vi "SwerveMain.vi"   [LabVIEW 2018]
uses:
  <vilib>/Rock Robotics/WPI/ThirdParty/Phoenix-LabVIEW/Motor Controller/Controls/CTRE_Phoenix_MotorControl_ControlMode.ctl
  <vilib>/Rock Robotics/Network Tables/NT Read Numeric Array.vi
  <vilib>/Rock Robotics/Network Tables/NT Write Numeric Array.vi
types:
  T1 = typedef "WPI_MotorControlDeviceRef.ctl" = cluster{"DeviceStatus":errorcluster, "Type":T2, "PWM":cluster{"PWM Channel":T3, "DeadBand":T4}, "CAN":cluster{"Device Number":u8, "SetOutput VI Ref":variant, "GetOutput VI Ref":variant, "Enable VI Ref":variant, "Disable VI Ref":variant, "Data":variant}, "Invert":bool, "DIO PWM":cluster{"PWM \"Enable\" Channel":T3, "DIOChannel":T5, "PWM Rate":dbl}}
  T2 = typedef "WPI_MotorControlType.ctl" = enum16{"PWM", "CAN", "DIO PWM"}
  T3 = typedef "FPGA_DIOPWMChannel.ctl" = enum8{"PWM 0", "PWM 1", "PWM 2", "PWM 3", "PWM 4", "PWM 5", "PWM 6", "PWM 7", "PWM 8", "PWM 9", "PWM MXP 0", "PWM MXP 1", "PWM MXP 2", "PWM MXP 3", "PWM MXP 4", "PWM MXP 5", "PWM MXP 6", "PWM MXP 7", "PWM MXP 8", "PWM MXP 9", "Invalid"}
  T4 = typedef "WPI_PWMDeadband.ctl" = cluster{"Name":string, "maxPositivePwm":i32, "minPositivePwm":i32, "centerPwm":i32, "maxNegativePwm":i32, "minNegativePwm":i32, "angularRange":u16}
  T5 = typedef "FPGA_DIOChannel.ctl" = enum8{"DIO 0", "DIO 1", "DIO 2", "DIO 3", "DIO 4", "DIO 5", "DIO 6", "DIO 7", "DIO 8", "DIO 9", "DIO MXP 0", "DIO MXP 1", "DIO MXP 2", "DIO MXP 3", "DIO MXP 4", "DIO MXP 5", "DIO MXP 6", "DIO MXP 7", "DIO MXP 8", "DIO MXP 9", "DIO MXP 10", "DIO MXP 11", "DIO MXP 12", "DIO MXP 13", "DIO MXP 14", "DIO MXP 15", "SPI Port CS1", "SPI Port CS2", "SPI Port CS3", "SPI Port MISO", "SPI Port MOSI", "Invalid"}
  T6 = typedef "WPI_AnalogChannelDevRef.ctl" = cluster{"DevStatus":errorcluster, "Analog Channel":T7}
  T7 = typedef "FPGA_AIChannel.ctl" = enum8{"AI 0", "AI 1", "AI 2", "AI 3", "AI MXP 0", "AI MXP 1", "AI MXP 2", "AI MXP 3", "Invalid"}
  T8 = cluster{"PhoenixMotorControlDevRef":T1, "PhoenixMotorControlDevRef":T1, "PhoenixMotorControlDevRef":T1, "PhoenixMotorControlDevRef":T1}
  T9 = typedef "CTRE_Phoenix_MotorControl_ControlMode.ctl" = u16
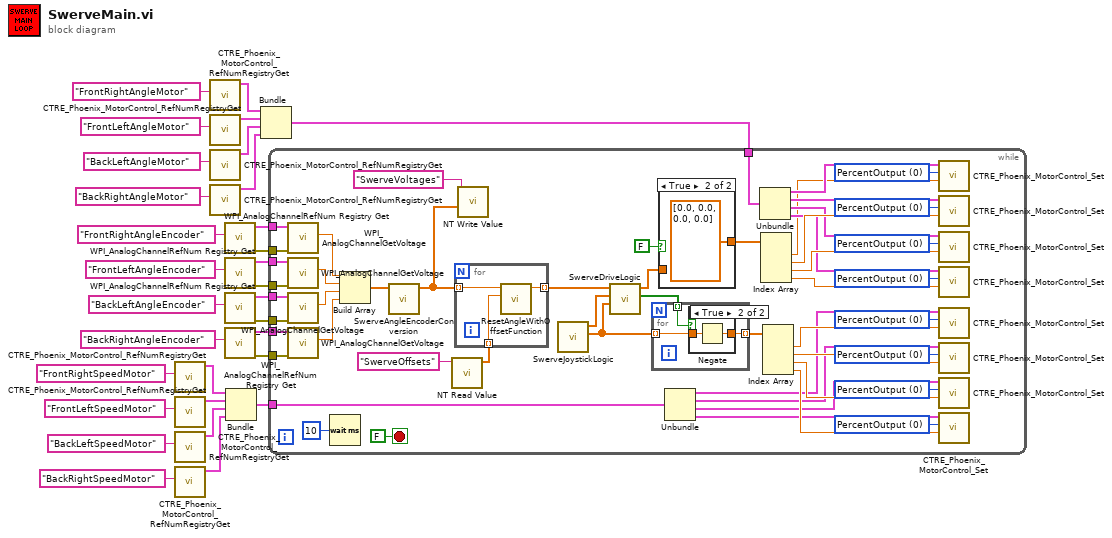
[diagram p0: block diagram]
diagram:
  n1 = call <vilib>:"CTRE_Phoenix_MotorControl_RefNumRegistryGet.vi"("refnum name"="FrontRightSpeedMotor") -> ("PhoenixMotorControlDevRef"=w8:T1)  [unwired: 9 in, 1 out]
  n2 = call <vilib>:"CTRE_Phoenix_MotorControl_RefNumRegistryGet.vi"("refnum name"="FrontLeftSpeedMotor") -> ("PhoenixMotorControlDevRef"=w16:T1)  [unwired: 9 in, 1 out]
  n3 = call <vilib>:"CTRE_Phoenix_MotorControl_RefNumRegistryGet.vi"("refnum name"="BackLeftSpeedMotor") -> ("PhoenixMotorControlDevRef"=w17:T1)  [unwired: 9 in, 1 out]
  n4 = call <vilib>:"CTRE_Phoenix_MotorControl_RefNumRegistryGet.vi"("refnum name"="BackRightSpeedMotor") -> ("PhoenixMotorControlDevRef"=w18:T1)  [unwired: 9 in, 1 out]
  n5 = call <vilib>:"CTRE_Phoenix_MotorControl_RefNumRegistryGet.vi"("refnum name"="FrontRightAngleMotor") -> ("PhoenixMotorControlDevRef"=w5:T1)  [unwired: 9 in, 1 out]
  n6 = call <vilib>:"CTRE_Phoenix_MotorControl_RefNumRegistryGet.vi"("refnum name"="FrontLeftAngleMotor") -> ("PhoenixMotorControlDevRef"=w9:T1)  [unwired: 9 in, 1 out]
  n7 = call <vilib>:"CTRE_Phoenix_MotorControl_RefNumRegistryGet.vi"("refnum name"="BackLeftAngleMotor") -> ("PhoenixMotorControlDevRef"=w10:T1)  [unwired: 9 in, 1 out]
  n8 = call <vilib>:"CTRE_Phoenix_MotorControl_RefNumRegistryGet.vi"("refnum name"="BackRightAngleMotor") -> ("PhoenixMotorControlDevRef"=w7:T1)  [unwired: 9 in, 1 out]
  n9 = call <vilib>:"WPI_AnalogChannelRefNum Registry Get.vi"("refnum name"="FrontRightAngleEncoder") -> ("error out"=w4:errorcluster, "AIDeviceRef"=w14:T6)  [unwired: 9 in]
  n10 = call <vilib>:"WPI_AnalogChannelRefNum Registry Get.vi"("refnum name"="FrontLeftAngleEncoder") -> ("error out"=w3:errorcluster, "AIDeviceRef"=w13:T6)  [unwired: 9 in]
  n11 = call <vilib>:"WPI_AnalogChannelRefNum Registry Get.vi"("refnum name"="BackLeftAngleEncoder") -> ("error out"=w2:errorcluster, "AIDeviceRef"=w12:T6)  [unwired: 9 in]
  n12 = call <vilib>:"WPI_AnalogChannelRefNum Registry Get.vi"("refnum name"="BackRightAngleEncoder") -> ("error out"=w1:errorcluster, "AIDeviceRef"=w11:T6)  [unwired: 9 in]
  n13 = Bundle("PhoenixMotorControlDevRef"=w8, "PhoenixMotorControlDevRef"=w16, "PhoenixMotorControlDevRef"=w17, "PhoenixMotorControlDevRef"=w18) -> (w15:T8)  [unwired: 1 in]
  n14 = Bundle("PhoenixMotorControlDevRef"=w5, "PhoenixMotorControlDevRef"=w9, "PhoenixMotorControlDevRef"=w10, "PhoenixMotorControlDevRef"=w7) -> (w6:T8)  [unwired: 1 in]
  n15 = while {
    tunnel: w15 -> [w34]
    tunnel: w14 -> [w83]
    tunnel: w13 -> [w82]
    tunnel: w12 -> [w81]
    tunnel: w11 -> [w80]
    tunnel: w6 -> [w33]
    tunnel: w4 -> [w41]
    tunnel: w3 -> [w40]
    tunnel: w2 -> [w39]
    tunnel: w1 -> [w38]
    stop <- FALSE stop-if-true
    w44 = T9 0 items=["PercentOutput"=0, "Position"=1, "Velocity"=2, "Current"=3, "Follower"=5, "MotionProfile"=6, "MotionMagic"=7, "MotionProfileArc"=10, "Disabled"=15] ("Control Mode")
    w45 = T9 0 items=["PercentOutput"=0, "Position"=1, "Velocity"=2, "Current"=3, "Follower"=5, "MotionProfile"=6, "MotionMagic"=7, "MotionProfileArc"=10, "Disabled"=15] ("Control Mode")
    w46 = T9 0 items=["PercentOutput"=0, "Position"=1, "Velocity"=2, "Current"=3, "Follower"=5, "MotionProfile"=6, "MotionMagic"=7, "MotionProfileArc"=10, "Disabled"=15] ("Control Mode")
    w47 = T9 0 items=["PercentOutput"=0, "Position"=1, "Velocity"=2, "Current"=3, "Follower"=5, "MotionProfile"=6, "MotionMagic"=7, "MotionProfileArc"=10, "Disabled"=15] ("Control Mode")
    w48 = T9 0 items=["PercentOutput"=0, "Position"=1, "Velocity"=2, "Current"=3, "Follower"=5, "MotionProfile"=6, "MotionMagic"=7, "MotionProfileArc"=10, "Disabled"=15] ("Control Mode")
    w49 = T9 0 items=["PercentOutput"=0, "Position"=1, "Velocity"=2, "Current"=3, "Follower"=5, "MotionProfile"=6, "MotionMagic"=7, "MotionProfileArc"=10, "Disabled"=15] ("Control Mode")
    w50 = T9 0 items=["PercentOutput"=0, "Position"=1, "Velocity"=2, "Current"=3, "Follower"=5, "MotionProfile"=6, "MotionMagic"=7, "MotionProfileArc"=10, "Disabled"=15] ("Control Mode")
    w51 = T9 0 items=["PercentOutput"=0, "Position"=1, "Velocity"=2, "Current"=3, "Follower"=5, "MotionProfile"=6, "MotionMagic"=7, "MotionProfileArc"=10, "Disabled"=15] ("Control Mode")
    n16 = call <vilib>:"WPI_AnalogChannelGetVoltage.vi"("error in (no error)"=w41, "AIDeviceRef"=w83) -> ("Voltage"=w79:dbl)  [unwired: 7 in, 2 out]
    n17 = call <vilib>:"WPI_AnalogChannelGetVoltage.vi"("error in (no error)"=w40, "AIDeviceRef"=w82) -> ("Voltage"=w78:dbl)  [unwired: 7 in, 2 out]
    n18 = call <vilib>:"WPI_AnalogChannelGetVoltage.vi"("error in (no error)"=w39, "AIDeviceRef"=w81) -> ("Voltage"=w77:dbl)  [unwired: 7 in, 2 out]
    n19 = call <vilib>:"WPI_AnalogChannelGetVoltage.vi"("error in (no error)"=w38, "AIDeviceRef"=w80) -> ("Voltage"=w76:dbl)  [unwired: 7 in, 2 out]
    n20 = Wait (ms)(milliseconds to wait=u32 10) -> ()  [unwired: 1 out]
    n21 = Build Array(w79, w78, w77, w76) -> (w32:dbl[])
    n22 = call "SwerveAngleEncoderConversion.vi"("Voltages"=w32) -> ("Angles"=w31:dbl[])  [unwired: 10 in]
    n23 = call-poly <vilib>:"NT Read Value.vi"("Name"="SwerveOffsets") -> ("Numeric Array"=w35:dbl[])  [unwired: 9 in, 1 out]
    n24 = for {
      tunnel: w31 -> [w86] mode=indexing
      tunnel: w35 -> [w88] mode=indexing
      tunnel: [w87] -> w59 mode=indexing
      n25 = call "ResetAngleWithOffsetFunction.vi"("Offset"=w88, "AngleInput"=w86) -> ("AngleOutput"=w87:dbl)  [unwired: 9 in]
    }
    n26 = call-poly <vilib>:"NT Write Value.vi"("Numeric Array"=w31, "Name"="SwerveVoltages") -> ()  [unwired: 9 in, 1 out]
    n27 = call "SwerveJoystickLogic.vi"() -> ("Speeds"=w55:dbl[], "Angles"=w58:dbl[])  [unwired: 9 in]
    n28 = call "SwerveDriveLogic.vi"("Speeds"=w55, "AngleSetpoints"=w58, "AngleEncoders"=w59) -> ("AngleMotorsReversed"=w60:bool[], "AngleMotorOutputs"=w57:dbl[])  [unwired: 7 in]
    n29 = for {
      tunnel: w55 -> [w90] mode=indexing
      tunnel: [w91] -> w68 mode=indexing
      tunnel: w60 -> [w89] mode=indexing
      n30 = case shown="True" w89 {
        tunnel: w90 -> [w92 w94]
        tunnel: [w92 w93] -> w91
        frame False {
        }
        frame True {
          n31 = Negate(x=w94) -> (-x=w93:dbl)
        }
      }
    }
    n32 = case shown="True" FALSE {
      tunnel: w57 -> [w84 _]
      tunnel: [w84 dbl[] [0.0, 0.0, 0.0, 0.0]] -> w56
      frame False {
      }
      frame True {
      }
    }
    n33 = Unbundle(w34) -> ("PhoenixMotorControlDevRef"=w53:T1, "PhoenixMotorControlDevRef"=w64:T1, "PhoenixMotorControlDevRef"=w63:T1, "PhoenixMotorControlDevRef"=w62:T1)
    n34 = Unbundle(w33) -> ("PhoenixMotorControlDevRef"=w71:T1, "PhoenixMotorControlDevRef"=w70:T1, "PhoenixMotorControlDevRef"=w69:T1, "PhoenixMotorControlDevRef"=w61:T1)
    n35 = Index Array(array=w56) -> (element #1=w43:dbl, element #2=w74:dbl, element #3=w73:dbl, element #4=w72:dbl)  [unwired: 4 in]
    n36 = Index Array(array=w68) -> (element #1=w54:dbl, element #2=w66:dbl, element #3=w65:dbl, element #4=w67:dbl)  [unwired: 4 in]
    n37 = call <vilib>:"CTRE_Phoenix_MotorControl_Set.vi"("Output"=w43, "Control Mode"=w51, "PhoenixMotorControlDevRef"=w71) -> ()  [unwired: 6 in, 3 out]
    n38 = call <vilib>:"CTRE_Phoenix_MotorControl_Set.vi"("Output"=w74, "Control Mode"=w50, "PhoenixMotorControlDevRef"=w70) -> ()  [unwired: 6 in, 3 out]
    n39 = call <vilib>:"CTRE_Phoenix_MotorControl_Set.vi"("Output"=w73, "Control Mode"=w49, "PhoenixMotorControlDevRef"=w69) -> ()  [unwired: 6 in, 3 out]
    n40 = call <vilib>:"CTRE_Phoenix_MotorControl_Set.vi"("Output"=w72, "Control Mode"=w48, "PhoenixMotorControlDevRef"=w61) -> ()  [unwired: 6 in, 3 out]
    n41 = call <vilib>:"CTRE_Phoenix_MotorControl_Set.vi"("Output"=w54, "Control Mode"=w47, "PhoenixMotorControlDevRef"=w53) -> ()  [unwired: 6 in, 3 out]
    n42 = call <vilib>:"CTRE_Phoenix_MotorControl_Set.vi"("Output"=w66, "Control Mode"=w46, "PhoenixMotorControlDevRef"=w64) -> ()  [unwired: 6 in, 3 out]
    n43 = call <vilib>:"CTRE_Phoenix_MotorControl_Set.vi"("Output"=w65, "Control Mode"=w45, "PhoenixMotorControlDevRef"=w63) -> ()  [unwired: 6 in, 3 out]
    n44 = call <vilib>:"CTRE_Phoenix_MotorControl_Set.vi"("Output"=w67, "Control Mode"=w44, "PhoenixMotorControlDevRef"=w62) -> ()  [unwired: 6 in, 3 out]
  }
